vi "Logging_Data.vi"(11 "Drive Loop Cluster":T3) -> (3 "Logging Data":T1)   [LabVIEW 2016]
doc: "Help file written by FRC Team 836 - The RoboBees\n\nThis VI writes the drive command, desired angle, and desired encoder values\nto the Logging Data control.\n\nThe Logging Data RT FIFO must be intialized using the \"Drive_Loop_Initialize_w_Help\" VI."
uses:
  <userlib>/836-Libraries/Drive/Drive_Code/Drive_Code_Support/Drive_Code_Bundle.ctl
  <userlib>/836-Libraries/Drive/Drive_Code/Drive_Code_Support/Sensor_Cluster.ctl
  <userlib>/836-Libraries/Drive/Drive_Code/Drive_Code_Support/Camera_Cluster.ctl
  <userlib>/836-Libraries/Drive/Drive_Code/Drive_Code_Support/Drive_Code_Notifier.ctl
  <userlib>/836-Libraries/Drive/Drive_Code/Drive_Code_Support/Drive_Code_Command.ctl
  <userlib>/836-Libraries/Drive/Drive_Code/Logging_Data.ctl
  <userlib>/836-Libraries/Drive/Drive_Code/Drive_Code_Support/Drive_Code_PID_Bundle.ctl
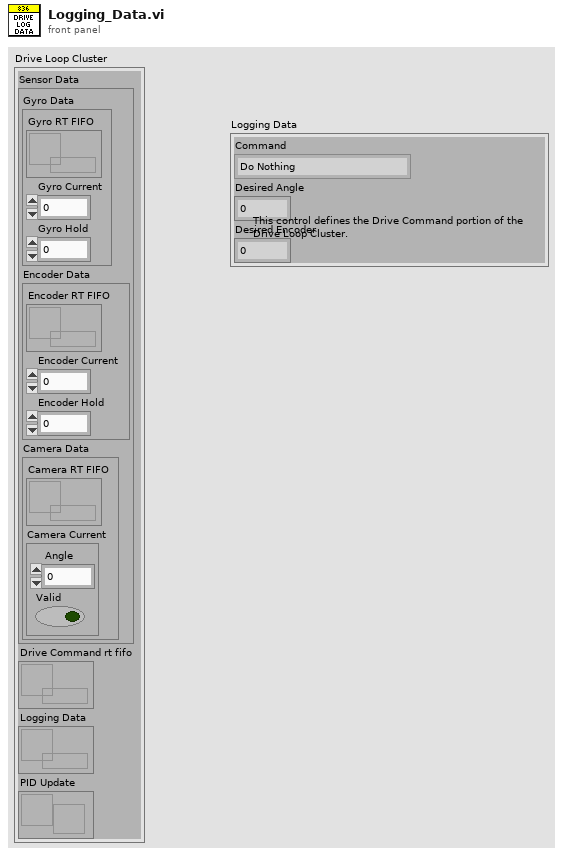
[diagram p1: front panel]
types:
  T1 = typedef "Logging_Data.ctl" = cluster{"Command":T2, "Desired Angle":dbl, "Desired Encoder":dbl}
  T2 = typedef "Drive_Code_Command.ctl" = enum16{"Do Nothing", "Manual", "Drive Continuous", "Turn", "Drive Distance", "Hold Position", "Hold Yaw", "Follow Camera", "Turn to Camera", "Approach Camera"}
  T3 = typedef "Drive_Code_Bundle.ctl" = cluster{"Sensor Data":T4, "Drive Command rt fifo":refnum<k33>, "Logging Data":refnum<k33>, "PID Update":refnum<notifier>}
  T4 = typedef "Sensor_Cluster.ctl" = cluster{"Gyro Data":cluster{"Gyro RT FIFO":refnum<k33>, "Gyro Current":dbl, "Gyro Hold":dbl}, "Encoder Data":cluster{"Encoder RT FIFO":refnum<k33>, "Encoder Current":dbl, "Encoder Hold":dbl}, "Camera Data":cluster{"Camera RT FIFO":refnum<k33>, "Camera Current":T5}}
  T5 = typedef "Camera_Cluster.ctl" = cluster{" Angle":dbl, "Valid":bool}
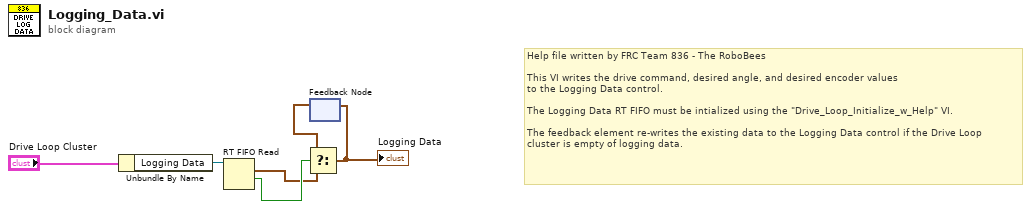
[diagram p0: block diagram]
diagram:
  # "Help file written by FRC Team 836 - The RoboBees\n\nThis VI writes the drive command, desired angle, and desired encoder values\nto the Logging Data control.\n\nThe Logging Data RT FIFO must be intialized using the \"Drive_Loop_Initialize_w_Help\" VI.\n\nThe feedback element re-writes the existing data to the Logging Data control if the Drive Loop\ncluster is empty of logging data."
  n1 = Unbundle By Name("Drive Loop Cluster") -> ("Logging Data"=w5:refnum<k33>)
  n2 = RT FIFO Read(0:w5) -> (9:w3:T1, 10:w4:bool)  [unwired: 3 in, 3 out]
  n3 = feedback #1() -> (w1:T1)  [unwired: 1 in]
  n4 = Select(t=w1, s=w4, f=w3) -> (s? t:f=w2:T1)
  "Logging Data" <- w2
  n5 = feedback-in #1(w2) -> ()
